vi "Plugins.vi"() -> (3 "Array":refnum<class "Dependency Source.lvclass">[](array[class]))   [LabVIEW 2019]
uses:
  Build/Project.Dependencies Finder.lvlibp/Dependency Source/Dependency Source.lvclass
  Build/Project.Dependencies Finder.lvlibp/Dependency Source_VIPM/Dependency Source_VIPM.lvclass
  C:/Current projects/LV32.2019..ProjectDependenciesFinder/Build/Project.Dependencies Finder.lvlibp/Dependency Source/Dependency Source.lvclass
  Build/Project.Dependencies Finder.lvlibp/Dependency Source_NIPM/Dependency Source_NIPM.lvclass
  Build/Project.Dependencies Finder.lvlibp/Dependency Source_GPM/Dependency Source_GPM.lvclass
  Build/Project.Dependencies Finder.lvlibp/Dependency Source_Custom/Dependency Source_Custom.lvclass
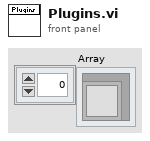
[diagram p1: front panel]
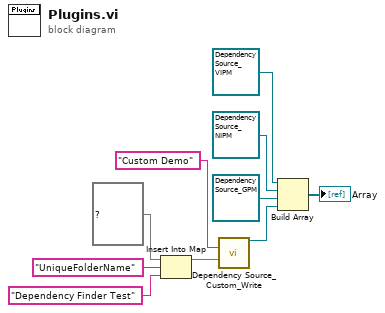
[diagram p0: block diagram]
diagram:
  n1 = Insert Into Map(map in=map{string, string} {} ("External Target Map"), key="UniqueFolderName", value="Dependency Finder Test") -> (map out=w8:map{string, string})  [unwired: 2 out]
  n2 = call "Dependency Source_Custom_Write.vi"("Dependency Source Name"="Custom Demo", "External Target Map"=w8) -> ("Dependency Source_Custom out"=w5:refnum<class "Dependency Source_Custom.lvclass">)  [unwired: 12 in, 1 out]
  n3 = Build Array(refnum<class "Dependency Source_VIPM.lvclass"> refnum ("Project.Dependencies Finder.lvlibp:Dependency Source_VIPM.lvclass"), refnum<class "Dependency Source_NIPM.lvclass"> refnum ("Project.Dependencies Finder.lvlibp:Dependency Source_NIPM.lvclass"), refnum<class "Dependency Source_GPM.lvclass"> refnum ("Project.Dependencies Finder.lvlibp:Dependency Source_GPM.lvclass"), w5) -> (→"Array":refnum<class "Dependency Source.lvclass">[])
